vi "Runden.vi"(8 "error in (no error)":errorcluster caption="Fehler (Eingang, kein Fehler)", 9 "Wert":dbl format="%#.15g", 11 "Stellen":i32) -> (0 "error out":errorcluster caption="Fehler (Ausgang)", 1 "gerundeter Wert":dbl format="%#.15g")   [LabVIEW 2020, in "allgemeine Sub-VIs.lvlib"]
uses:
  allgemeine Sub-VIs.lvlib
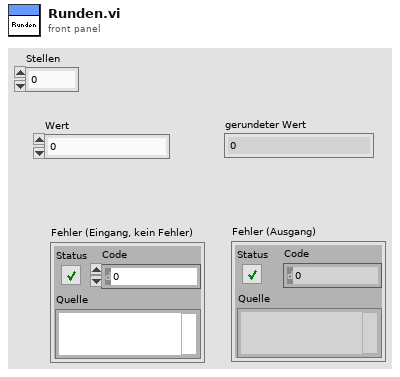
[diagram p1: front panel]
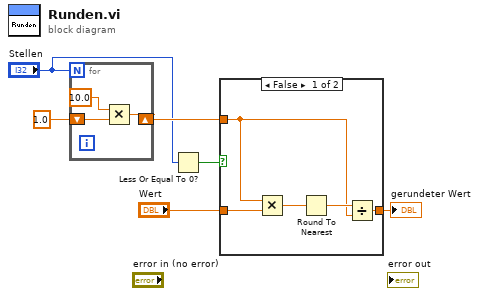
[diagram p0: block diagram]
diagram:
  n1 = for {
    N: "Stellen" -> [_]
    shift-right: [w7] -> w4
    shift-left: 1.0 -> [w9]
    n2 = Multiply(x=10.0, y=w9) -> (x*y=w7:dbl)
  }
  n3 = Less Or Equal To 0?(x="Stellen") -> (x <= 0?=w1:bool)
  n4 = case shown="False" w1 {
    tunnel: "Wert" -> [w14 w15]
    tunnel: w4 -> [w11 _]
    tunnel: [w10 w15] -> w3
    frame False {
      n5 = Multiply(x=w11, y=w14) -> (x*y=w13:dbl)
      n6 = Round To Nearest(number=w13) -> (nearest integer value=w12:dbl)
      n7 = Divide(x=w12, y=w11) -> (x/y=w10:dbl)
    }
    frame True {
    }
  }
  "gerundeter Wert" <- w3
